vi "MCP4725 Generate and Read Example 2.vi"(8 "Error In":errorcluster) -> (0 "Error Out":errorcluster)   [LabVIEW 2014]
doc: "This example produces stepped triangle wave on output in loop, there's no timing inside while loop so it's running as fast as it can, at test computer signal has frequency 440Hz and consists from 12 samples, so we are able to produce this fast signals at most."
uses:
  LabVIEW-Universal-Transcriptor-MCP4725/MCP4725.lvclass
  <vilib>/LabVIEW Universal Transcriptor/LabVIEW to Arduino Transcriptor/Transcriptors/System API/Serial println string.vi
panel:
  # "This example produces stepped triangle wave on output in loop, there's no timing inside while loop so it's running as fast as it can, at test computer signal has frequency 440Hz and consists from 12 samples, so we are able to produce this fast signals at most.\n\nWiring:\n  Arduino Nano  |  MCP4725 module\n  -----------------------------------------\n          VCC        |           +5V\n          GND        |           GND\n          A4           |           SDA\n          A5           |           SCL"
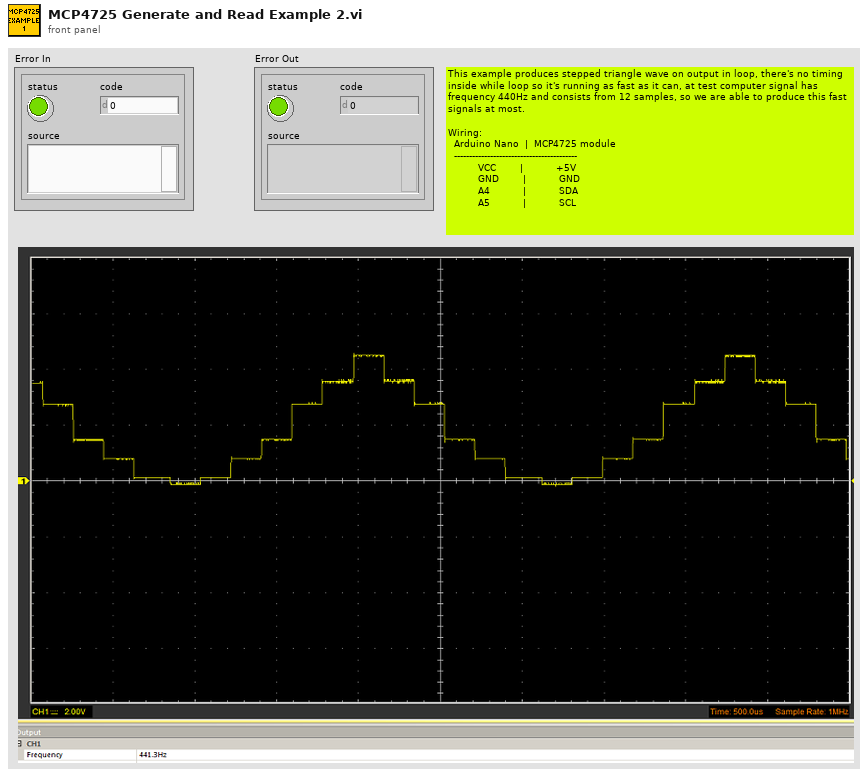
[diagram p1: front panel]
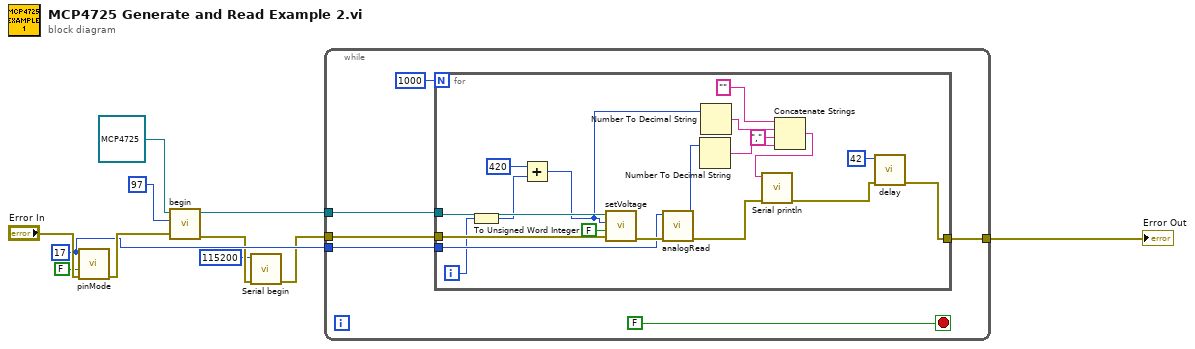
[diagram p0: block diagram]
diagram:
  w4 = 17 ("pin number")
  n1 = call <vilib>:"pinMode.vi"("Error In"="Error In", "output?"=FALSE, "pin number"=w4) -> ("Error Out"=w6:errorcluster)  [unwired: 8 in]
  n2 = call "begin.vi"("error in (no error)"=w6, "I2C addr"=u8 97, "MCP4725 in"=refnum<class "MCP4725.lvclass"> refnum) -> ("error out"=w3:errorcluster, "MCP4725 out"=w10:refnum<class "MCP4725.lvclass">)  [unwired: 7 in]
  n3 = call <vilib>:"Serial begin.vi"("Error In"=w3, "speed (Bd)"=115200) -> ("Error Out"=w2:errorcluster)  [unwired: 9 in]
  n4 = while {
    tunnel: w2 -> [w16]
    tunnel: w10 -> [w15]
    tunnel: [w14] -> w9
    tunnel: w4 -> [w13]
    stop <- FALSE stop-if-true
    n5 = for {
      N: 1000 -> [_]
      tunnel: w16 -> [w36]
      tunnel: w15 -> [w35]
      tunnel: [w22] -> w14
      tunnel: w13 -> [w32]
      i -> [w24]
      n6 = To Unsigned Word Integer(number=w24) -> (unsigned 16bit integer=w19:u16)
      n7 = Add(x=u16 420, y=w19) -> (x+y=w18:u16)
      n8 = call "setVoltage.vi"("error in (no error)"=w36, "writeEEPROM?"=FALSE, "voltage"=w18, "MCP4725 in"=w35) -> ("error out"=w33:errorcluster)  [unwired: 6 in, 1 out]
      n9 = call <vilib>:"analogRead.vi"("Error In"=w33, "pin number"=w32) -> ("Error Out"=w31:errorcluster, "value"=w30:u16)  [unwired: 8 in]
      n10 = Number To Decimal String(number=w30) -> (decimal integer string=w27:string)  [unwired: 1 in]
      n11 = Number To Decimal String(number=w18) -> (decimal integer string=w29:string)  [unwired: 1 in]
      n12 = Concatenate Strings("" ("string"), w29, "," ("string"), w27) -> (w25:string)
      n13 = call-poly <vilib>:"Serial println.vi"("Error In"=w31, "string in"=w25) -> ("Error Out"=w23:errorcluster)  [unwired: 9 in]
      n14 = call <vilib>:"delay.vi"("Error In"=w23, "time (ms)"=42) -> ("Error Out"=w22:errorcluster)  [unwired: 9 in]
    }
  }
  "Error Out" <- w9
